vi "题目六.vi"   [LabVIEW 2017]
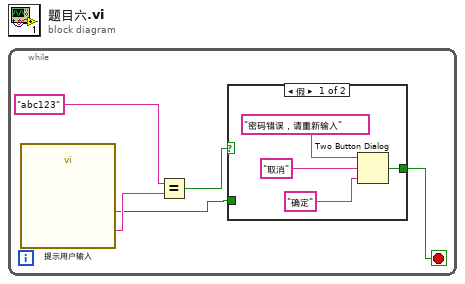
[diagram p0: block diagram]
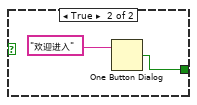
[diagram p2: hidden frame]
diagram:
  n1 = while {
    stop <- w1 stop-if-true
    n2 = call "提示用户输入"() -> ("请输入密码"=w5:string, "确定"=w2:bool)  [unwired: 17 in, 1 out]
    n3 = Equal?(x="abc123", y=w5) -> (x = y?=w3:bool)
    n4 = case shown="假" w3 {
      tunnel: w2 -> [_ _]
      tunnel: [w8 w10] -> w1
      frame False {
        n5 = Two Button Dialog(message="密码错误，请重新输入", 1:"确定", 2:"取消") -> (T button?=w8:bool)
      }
      frame True {
        n6 = One Button Dialog(message="欢迎进入") -> (true=w10:bool)  [unwired: 1 in]
      }
    }
  }
